vi "StartProgram.vi"(8 "error in (no error)":errorcluster, 10 "Номер банка программ":u16(ring) items=["0", "1", "2", "3", "4", "5", "6", "7"], 11 "StepMotor in":refnum<class "StepMotor.lvclass">) -> (0 "error out":errorcluster, 3 "StepMotor out":refnum<class "StepMotor.lvclass">)   [LabVIEW 2010, in "StepMotor.lvclass"]
uses:
  StepMotor.lvclass
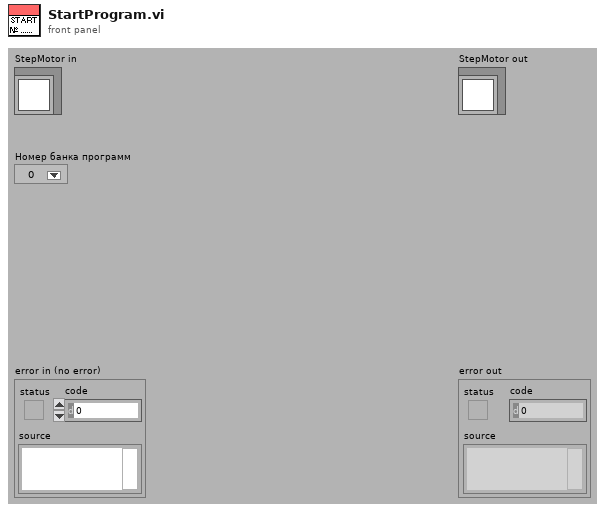
[diagram p1: front panel]
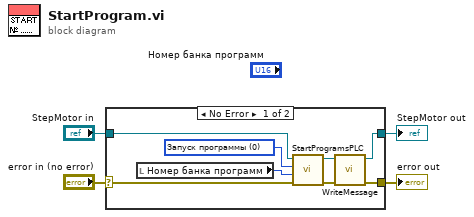
[diagram p0: block diagram]
diagram:
  n1 = case shown="No Error" "error in (no error)" {
    selector: "error in (no error)" -> [w5 w14]
    tunnel: [w7 w14] -> w3
    tunnel: [w8 w13] -> w1
    tunnel: "StepMotor in" -> [w6 w13]
    frame No Error {
      w10 = u16 0 items=["Запуск программы", "Останов текущей программы"] ("Адрес параметра")
      n2 = local read "Номер банка программ"() -> (w9:u16)
      n3 = call-dynamic "StartProgramsPLC.vi"("error in (no error)"=w5, "Номер банка программ"=w9, "Тип запроса"=w10, "StepMotor in"=w6) -> ("error out"=w12:errorcluster, "StepMotor out"=w11:refnum<class "StepMotor.lvclass">)  [unwired: 6 in]
      n4 = call-dynamic "WriteMessage.vi"("error in (no error)"=w12, "StepMotor in"=w11) -> ("error out"=w7:errorcluster, "StepMotor out"=w8:refnum<class "StepMotor.lvclass">)  [unwired: 8 in]
    }
    frame Error {
    }
  }
  "error out" <- w3
  "StepMotor out" <- w1
